vi "Execute.vi"(7 "Actor in":refnum<class "Actor.lvclass">, 8 "Error in":errorcluster, 11 "TEMPLATE Msg in":refnum<class "TEMPLATE Msg.lvclass">) -> (0 "Error out":errorcluster, 2 "Msg Output":refnum<class "Msg Output.lvclass">, 5 "Actor out":refnum<class "Actor.lvclass">)   [LabVIEW 2025, in "_Template.lvlib" / "Templates.lvlib" / "TEMPLATE jettl Msg.lvlib" / "TEMPLATE Msg.lvlib" / "TEMPLATE Msg.lvclass"]
uses:
  TEMPLATE Msg.lvclass
  jettl/jettl/Actor/Actor.lvclass
  jettl/jettl/Msg Output/Msg Output.lvclass
  TEMPLATE jettl Msg/TEMPLATE jettl Msg.lvclass
  TEMPLATE Msg.lvclass/TEMPLATE Msg.ctl
  TEMPLATE Msg Output/TEMPLATE Msg Output.lvlib
  TEMPLATE Msg Input/TEMPLATE Msg Input.lvlib
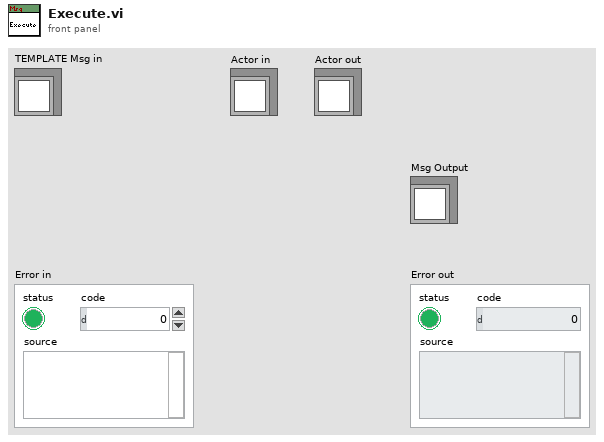
[diagram p1: front panel]
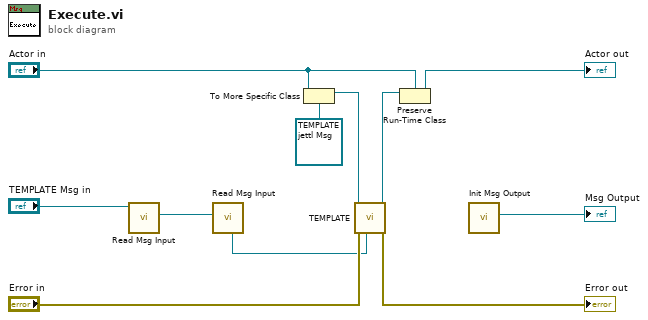
[diagram p0: block diagram]
diagram:
  n1 = call-dynamic "Read Msg Input.vi"("TEMPLATE Msg in"="TEMPLATE Msg in") -> ("Msg Input"=w1:refnum<class "Msg Input.lvclass">)  [unwired: 10 in]
  n2 = call "Read Msg Input.vi"("Msg Input"=w1) -> ("Teller"=w3:refnum<class "Teller.lvclass">)  [unwired: 10 in]
  n3 = To More Specific Class(target class=refnum<class "TEMPLATE jettl Msg.lvclass"> refnum ("jettl Msg Template"), reference="Actor in") -> (specific class reference=w10:refnum<class "TEMPLATE jettl Msg.lvclass">)  [unwired: 1 in, 1 out]
  n4 = call-dynamic "TEMPLATE.vi"("Teller"=w3, "Error in"="Error in", "TEMPLATE jettl Msg in"=w10) -> ("Error out"=→"Error out":errorcluster, "TEMPLATE jettl Msg out"=w9:refnum<class "TEMPLATE jettl Msg.lvclass">)  [unwired: 7 in]
  n5 = Preserve Run-Time Class(object in=w9, 2:"Actor in") -> (object out=→"Actor out":refnum<class "Actor.lvclass">)  [unwired: 1 in, 1 out]
  n6 = call "Init Msg Output.vi"() -> ("Msg Output"=→"Msg Output":refnum<class "Msg Output.lvclass">)  [unwired: 11 in]
